vi "3458A Utility Output Format.vi"(5 "Output Format (0:ASCII)":T1(ring), 7 "Numbers of Reading (1)":i32=1, 9 "Input String":string) -> (4 "Output Data (ASCII)":dbl[](array[numeric]) format="%.4e", 6 "Output Data (Double Real)":dbl[](array[numeric]) format="%.4e", 8 "Output Data (Single Real)":sgl[](array[numeric]) format="%.4e", 10 "Output Data (Single Integer)":i16[](array[numeric]), 13 "binary converted to int32":i32[](array[numeric]) format="%.4e", 14 "anything converted to double":dbl[](array[numeric]), 15 "Output Data (Double Integer)":i32[](array[numeric]) format="%.4e")   [LabVIEW 2013, in "3458A Virtual Digitizer.lvlib" / "3458A Digitizing Low Levels.lvlib"]
doc: "This VI takes an input string and converts the string into numeric value according to the type of data that are being sent back. If the data type is not in ASCII characters, typecasting is then performed to changes the string into numeric type, with each number stored as an element in the output array."
uses:
  3458A Digitizing Low Levels.lvlib
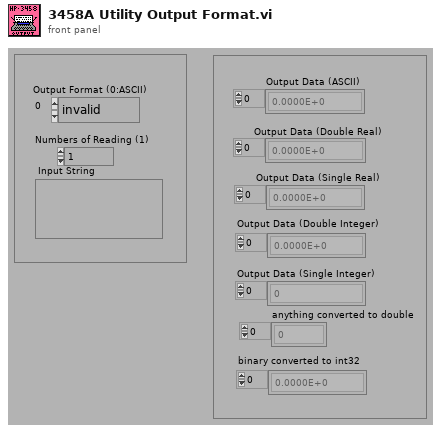
[diagram p1: front panel]
types:
  T1 = enum16{"invalid", "ASCII", "SINT", "DINT", "SREAL", "DREAL"}
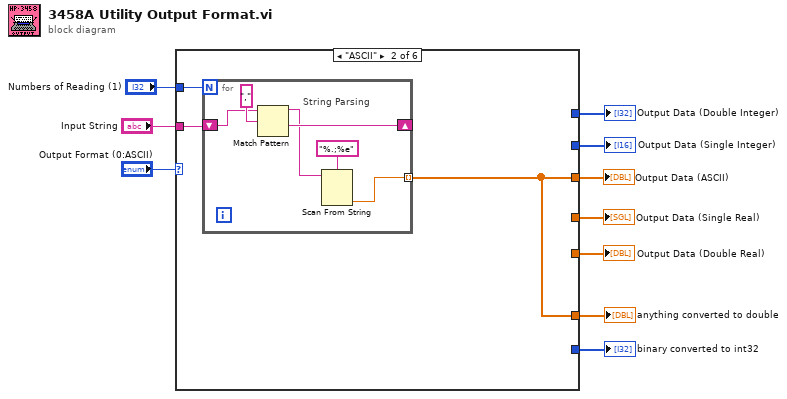
[diagram p0: block diagram]
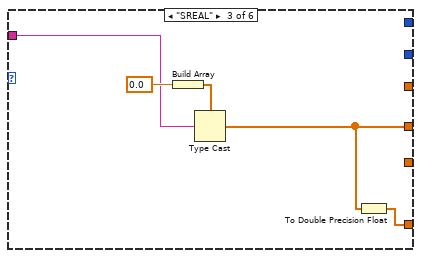
[diagram p3: hidden frame]
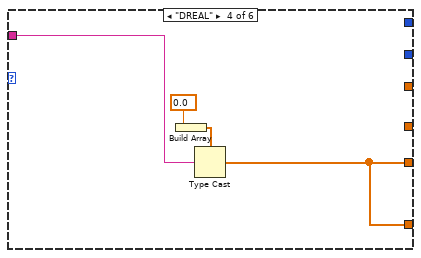
[diagram p4: hidden frame]
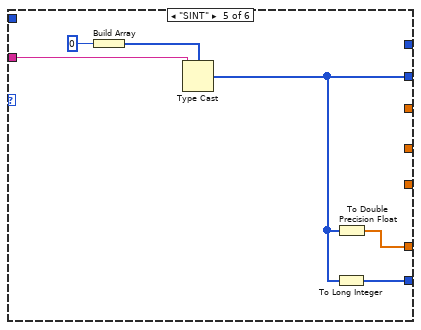
[diagram p5: hidden frame]
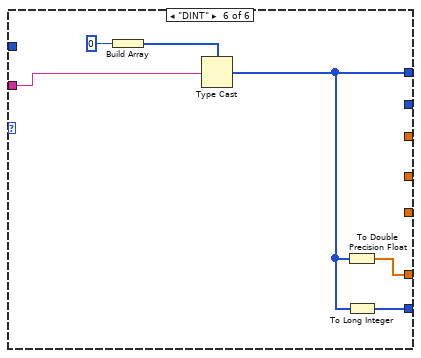
[diagram p6: hidden frame]
diagram:
  n1 = case shown="\"ASCII\"" "Output Format (0:ASCII)" {
    tunnel: [_ _ _ w25 _ _] -> w6
    tunnel: [_ _ w20 _ _ _] -> w7
    tunnel: [_ w11 _ _ _ _] -> w8
    tunnel: "Input String" -> [_ w12 w22 w26 w33 w38]
    tunnel: "Numbers of Reading (1)" -> [_ w13 _ _ _ _]
    tunnel: [_ _ _ _ w30 _] -> w4
    tunnel: [_ _ _ _ _ w36] -> w3
    tunnel: [_ w11 w21 w25 w31 w37] -> w2
    tunnel: [_ _ _ _ w29 w35] -> w1
    frame "invalid" {
    }
    frame "ASCII" {
      n2 = for {
        N: w13 -> [_]
        tunnel: [w18] -> w11 mode=indexing
        shift-right: [w16] -> _
        shift-left: w12 -> [w15]
        # "String Parsing"
        n3 = Match Pattern(string=w15, regular expression=",") -> (before substring=w14:string, after substring=w16:string)  [unwired: 1 in, 2 out]
        n4 = Scan From String(format string="%.;%e", input string=w14) -> (output 1=w18:dbl)  [unwired: 3 in, 3 out]
      }
    }
    frame "SREAL" {
      n5 = Build Array(sgl 0.0 ("single floating point representation")) -> (w24:sgl[])
      n6 = Type Cast(type=w24, x=w22) -> (*(type *) &x=w20:sgl[])
      n7 = To Double Precision Float(number=w20) -> (double precision float=w21:dbl[])
    }
    frame "DREAL" {
      n8 = Build Array(0.0 ("double floating point representation")) -> (w28:dbl[])
      n9 = Type Cast(type=w28, x=w26) -> (*(type *) &x=w25:dbl[])
    }
    frame "SINT" {
      n10 = Build Array(i16 0 ("word integer representation")) -> (w34:i16[])
      n11 = Type Cast(type=w34, x=w33) -> (*(type *) &x=w30:i16[])
      n12 = To Long Integer(number=w30) -> (32bit integer=w29:i32[])
      n13 = To Double Precision Float(number=w30) -> (double precision float=w31:dbl[])
    }
    frame "DINT" {
      n14 = Build Array(0 ("long integer representation")) -> (w40:i32[])
      n15 = Type Cast(type=w40, x=w38) -> (*(type *) &x=w36:i32[])
      n16 = To Double Precision Float(number=w36) -> (double precision float=w37:dbl[])
      n17 = To Long Integer(number=w36) -> (32bit integer=w35:i32[])
    }
  }
  "Output Data (ASCII)" <- w8
  "Output Data (Single Real)" <- w7
  "Output Data (Double Real)" <- w6
  "Output Data (Single Integer)" <- w4
  "Output Data (Double Integer)" <- w3
  "anything converted to double" <- w2
  "binary converted to int32" <- w1
